vi "VISAArray.vi"(10 "VISA Array In":refnum<visa-resource-name>[](array[refnum])) -> (2 "VISA Array Out":refnum<visa-resource-name>[](array[refnum]))   [LabVIEW 2013]
panel:
  out "Array 3":u64[](array[numeric])
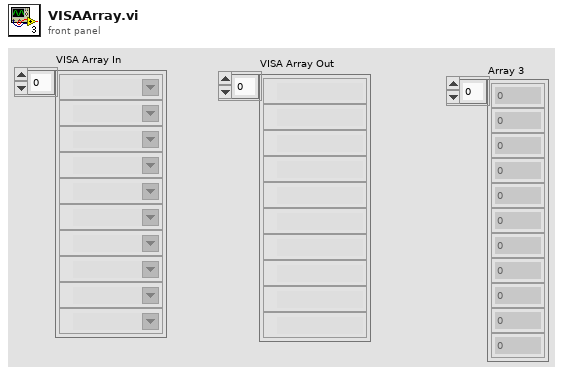
[diagram p1: front panel]
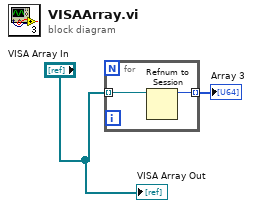
[diagram p0: block diagram]
diagram:
  n1 = for {
    tunnel: "VISA Array In" -> [w4] mode=indexing
    tunnel: [w3] -> w1 mode=indexing
    n2 = Refnum to Session(7:w4) -> (3:w3:u64)  [unwired: 1 in, 1 out]
  }
  "Array 3" <- w1
  "VISA Array Out" <- "VISA Array In"
